vi "Process.vi"(8 "error in (no error)":errorcluster, 10 "Pound in":refnum<class "Pound.lvclass">, 11 "Qbus in":refnum<class "Qbus.lvclass">) -> (0 "error out":errorcluster)   [LabVIEW 2017, in "BurstMode.lvlib"]
doc: "The Trigger process evaluates the expressions that define when a data group enters and exits operating states. After determining the current operating state of the data goup, this process evaluates the file-collection expression for that state to determine whether to collect a file."
uses:
  <vilib>/addons/InsightCM/Devices/Shared/Cms/CmsBurstMode/BurstMode.lvlib
  <vilib>/addons/Qbus/Qbus.lvclass
  <vilib>/NI/Software Watchdog/Pound/Pound.lvclass
  <vilib>/addons/InsightCM/Devices/Shared/Cms/CmsBurstMode/controls/config.ctl
  <vilib>/addons/TimerProcess/controls/taskType.ctl
  <vilib>/addons/InsightCM/Devices/Shared/Cms/CmsBurstMode/controls/BurstModeComplete.ctl
  <vilib>/NI/Software Watchdog/Watchdog/Watchdog.lvclass
  <vilib>/addons/TraceLogger/TraceLogger.lvlib
  <vilib>/addons/InsightCM/Devices/Shared/Common/ServerComm/ServerComm.lvlib
  <vilib>/addons/InsightCM/Devices/Shared/Common/DataFlow/DataFlow.lvlib
  <vilib>/addons/InsightCM/Utilities/GlobalConfiguration/GlobalConfiguration.lvlib
  <vilib>/addons/TimerProcess/TimerProcess.lvlib
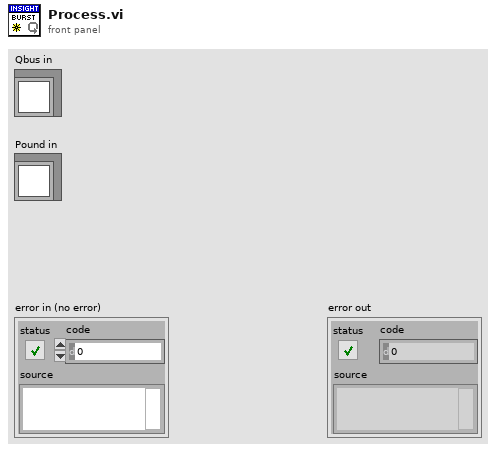
[diagram p1: front panel]
types:
  T1 = typedef "BurstMode.lvlib/config.ctl" = cluster{"Device":string, "Groups":string[], "ForceBurst":variant, "TriggerBurst":variant, "Burst Mode Count":i32, "Enabled":bool}
  T2 = typedef "TimerProcess.lvlib/taskType.ctl" = enum16{"single", "repeat"}
  T3 = typedef "BurstMode.lvlib/BurstModeComplete.ctl" = cluster{"Group":string}
  T4 = typedef "DataFlow.lvlib/Data.ctl" = cluster{"DataGroup":string, "Waveforms":T5, "Map":T6, "Type":T7}
  T5 = typedef "wfmSGL_DVR.ctl" = refnum<data-value>
  T6 = typedef "PointValueMap.lvlib/PointMap.ctl" = refnum<data-value>
  T7 = typedef "DataFlow.lvlib/Type.ctl" = enum16{"High Rate", "Low Rate", "Burst Mode"}
  T8 = typedef "Message.ctl" = cluster{"Header":T9, "Body":u8[]}
  T9 = typedef "MessageHeader.ctl" = cluster{"MessageName":string, "Timestamp":i64, "CorrelationId":string, "ContentType":string, "RoutingKey":string, "Properties":T10[]}
  T10 = typedef "KeyValuePair.ctl" = cluster{"Key":string, "Value":string}
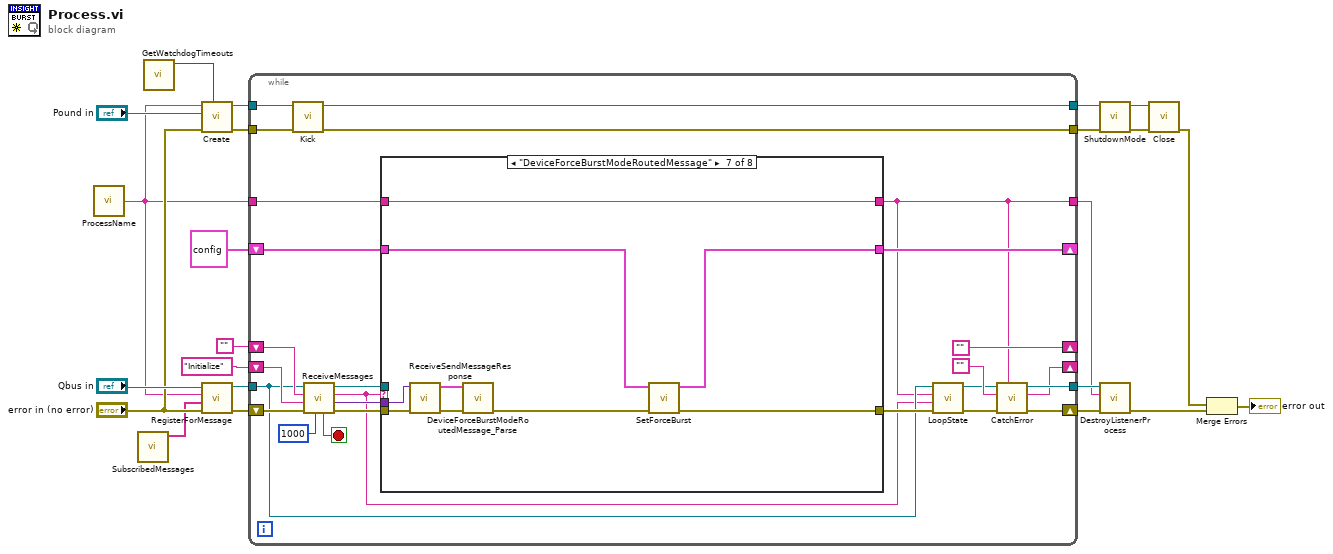
[diagram p0: block diagram]
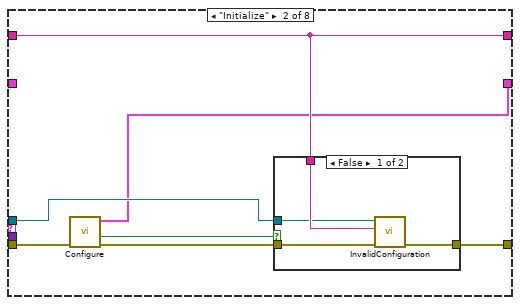
[diagram p3: hidden frame]
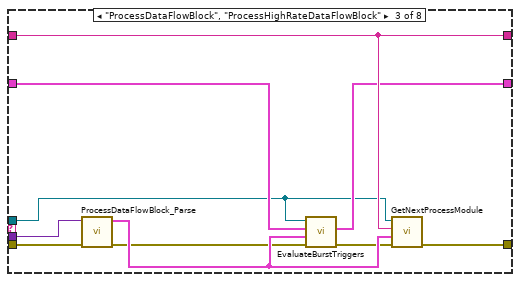
[diagram p5: hidden frame]
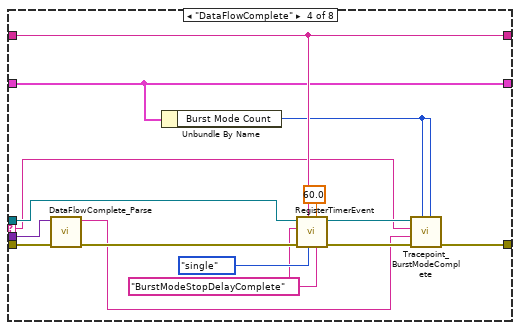
[diagram p6: hidden frame]
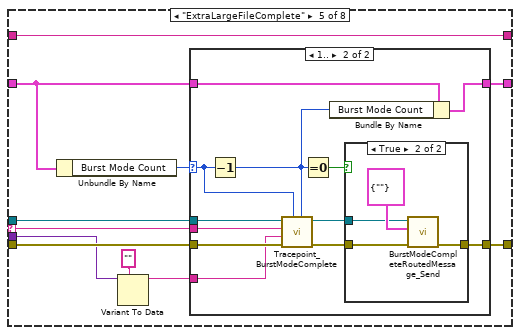
[diagram p7: hidden frame]
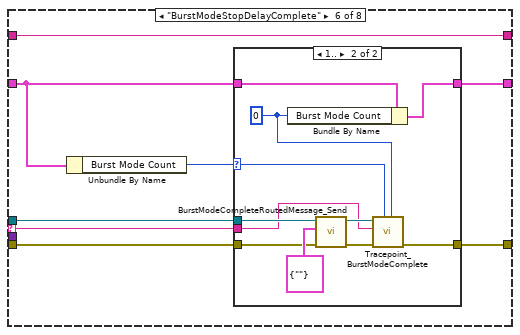
[diagram p10: hidden frame]
diagram:
  n1 = call <vilib>:"ProcessName.vi"() -> ("process name"=w3:string)  [unwired: 5 in]
  n2 = call <vilib>:"SubscribedMessages.vi"() -> ("subscribed messages"=w2:string[])  [unwired: 11 in]
  n3 = call <vilib>:"GetWatchdogTimeouts.vi"() -> ("software timeout"=w4:u32)  [unwired: 10 in, 1 out]
  n4 = call <vilib>:"Create.vi"("Execution Timeout (ms)"=w4, "error in (no error)"="error in (no error)", "Pound"="Pound in", "Name"=w3) -> ("error out"=w13:errorcluster, "Watchdog"=w12:refnum<data-value>)  [unwired: 6 in]
  n5 = call <vilib>:"RegisterForMessage.vi"("error in (no error)"="error in (no error)", "message names"=w2, "process name"=w3, "Qbus in"="Qbus in") -> ("error in (no error)"=w22:errorcluster, "Qbus out"=w21:refnum<class "Qbus.lvclass">)  [unwired: 6 in]
  n6 = while {
    shift-right: [""] -> _
    shift-left: "" -> [w47]
    tunnel: w21 -> [w33]
    tunnel: w3 -> [w35]
    tunnel: [w38] -> w18
    tunnel: [w28] -> w17
    shift-right: [w36] -> _
    shift-left: "Initialize" -> [w42]
    shift-right: [w40] -> _
    shift-left: T1 {"Device"="", "Groups"=[], "ForceBurst"=variant, "TriggerBurst"=variant, "Burst Mode Count"=0, "Enabled"=FALSE} ("config") -> [w41]
    tunnel: w13 -> [w32]
    tunnel: w12 -> [w31]
    tunnel: [w30] -> w8
    tunnel: [w29] -> w7
    shift-right: [w39] -> w20
    shift-left: w22 -> [w49]
    stop <- w48 stop-if-true
    n7 = call <vilib>:"Kick.vi"("error in (no error)"=w32, "Watchdog"=w31) -> ("error out"=w29:errorcluster, "Watchdog"=w30:refnum<data-value>)  [unwired: 8 in]
    n8 = call <vilib>:"ReceiveMessages.vi"("timeout (1000)"=1000 ("milliseconds to wait"), "error in (no error)"=w49, "priority action"=w42, "default action"=w47, "Qbus in"=w33) -> ("error out"=w46:errorcluster, "message value"=w43:variant, "action"=w27:string, "Qbus out"=w44:refnum<class "Qbus.lvclass">, "exit"=w48:bool)  [unwired: 2 in]
    n9 = case shown="\"DeviceForceBurstModeRoutedMessage\"" w27 {
      selector: w27 -> [_ _ _ w78 w95 w123 _ _]
      tunnel: w46 -> [w50 w56 w73 w88 w100 w126 w148 w150]
      tunnel: w44 -> [_ w59 w65 w87 w98 w124 _ _]
      tunnel: [w50 w58 w74 w79 w99 w125 w144 w150] -> w34
      tunnel: w43 -> [_ _ w72 w89 w92 _ w147 _]
      tunnel: w41 -> [w52 _ w70 w77 w96 w121 w146 w152]
      tunnel: [w52 w53 w69 w77 w97 w120 w145 w152] -> w40
      tunnel: [w51 w57 w71 w86 w93 w127 w149 w151] -> w28
      tunnel: w35 -> [w51 w57 w71 w86 w93 w127 w149 w151]
      frame "", Default {
      }
      frame "Initialize" {
        n10 = call <vilib>:"Configure.vi"("error in (no error)"=w56) -> ("error out"=w55:errorcluster, "valid configuration"=w54:bool, "config"=w53:T1)  [unwired: 8 in]
        n11 = case shown="False" w54 {
          tunnel: w59 -> [w61 _]
          tunnel: [w63 w64] -> w58
          tunnel: w55 -> [w60 w64]
          tunnel: w57 -> [w62 _]
          frame False {
            n12 = call <vilib>:"InvalidConfiguration.vi"("error in (no error)"=w60, "description"=w62, "Qbus in"=w61) -> ("error out"=w63:errorcluster)  [unwired: 7 in, 1 out]
          }
          frame True {
          }
        }
      }
      frame "ProcessDataFlowBlock", "ProcessHighRateDataFlowBlock" {
        n13 = call <vilib>:"ProcessDataFlowBlock_Parse.vi"("error in (no error)"=w73, "body"=w72) -> ("error out"=w67:errorcluster, "data"=w68:T4)  [unwired: 8 in]
        n14 = call <vilib>:"EvaluateBurstTriggers.vi"("error in (no error)"=w67, "data"=w68, "config"=w70, "Qbus in"=w65) -> ("error out"=w66:errorcluster, "config out"=w69:T1)  [unwired: 6 in]
        n15 = call <vilib>:"GetNextProcessModule.vi"("error in (no error)"=w66, "data"=w68, "source"=w71, "Qbus in"=w65) -> ("error out"=w74:errorcluster)  [unwired: 6 in, 1 out]
      }
      frame "DataFlowComplete" {
        w82 = "BurstModeStopDelayComplete" ("timer task name")
        n16 = call <vilib>:"DataFlowComplete_Parse.vi"("error in (no error)"=w88, "body"=w89) -> ("error out"=w85:errorcluster, "group"=w75:string)  [unwired: 8 in]
        n17 = Unbundle By Name(w77) -> ("Burst Mode Count"=w76:i32)
        n18 = call <vilib>:"RegisterTimerEvent.vi"("timer task name"=w82, "interval (sec)"=60.0, "type"=taskType."single", "process name"=w86, "error in (no error)"=w85, "callback action"=w82, "qbus in"=w87) -> ("error out"=w80:errorcluster, "qbus out"=w81:refnum<class "Qbus.lvclass">)  [unwired: 3 in]
        n19 = call <vilib>:"Tracepoint_BurstModeComplete.vi"("new count"=w76, "prev count"=w76, "error in (no error)"=w80, "group"=w75, "type"=w78, "Qbus"=w81) -> ("error out"=w79:errorcluster)  [unwired: 4 in, 1 out]
      }
      frame "ExtraLargeFileComplete" {
        n20 = Unbundle By Name(w96) -> ("Burst Mode Count"=w94:i32)
        n21 = Variant To Data(type="", Variant=w92) -> (data=w90:string)  [unwired: 1 in, 1 out]
        n22 = case shown="1.." w94 {
          selector: w94 -> [_ w104]
          tunnel: w100 -> [w101 w108]
          tunnel: [w101 w114] -> w99
          tunnel: w98 -> [_ w110]
          tunnel: w95 -> [_ w105]
          tunnel: w96 -> [w102 w112]
          tunnel: [w102 w111] -> w97
          tunnel: w90 -> [_ w106]
          frame 0, Default {
          }
          frame 1.. {
            n23 = Decrement(x=w104) -> (x-1=w103:i32)
            n24 = call <vilib>:"Tracepoint_BurstModeComplete.vi"("new count"=w103, "prev count"=w104, "error in (no error)"=w108, "group"=w106, "type"=w105, "Qbus"=w110) -> ("error out"=w107:errorcluster, "Qbus out"=w109:refnum<class "Qbus.lvclass">)  [unwired: 4 in]
            n25 = Equal To 0?(x=w103) -> (x = 0?=w113:bool)
            n26 = Bundle By Name(cluster=w112, "Burst Mode Count"=w103) -> (w111:T1)
            n27 = case shown="True" w113 {
              tunnel: w107 -> [w115 w118]
              tunnel: [w115 w116] -> w114
              tunnel: w109 -> [_ w117]
              frame False {
              }
              frame True {
                n28 = call <vilib>:"BurstModeCompleteRoutedMessage_Send.vi"("error in (no error)"=w118, "BurstModeComplete"=T3 {"Group"=""}, "Qbus in"=w117) -> ("error out"=w116:errorcluster)  [unwired: 7 in, 1 out]
              }
            }
          }
        }
      }
      frame "BurstModeStopDelayComplete" {
        n29 = Unbundle By Name(w121) -> ("Burst Mode Count"=w122:i32)
        n30 = case shown="1.." w122 {
          selector: w122 -> [_ w131]
          tunnel: w126 -> [w128 w138]
          tunnel: [w128 w137] -> w125
          tunnel: w124 -> [_ w136]
          tunnel: w123 -> [_ w134]
          tunnel: w121 -> [w129 w133]
          tunnel: [w129 w132] -> w120
          frame 0, Default {
          }
          frame 1.. {
            w130 = 0 ("Burst Mode Count")
            n31 = Bundle By Name(cluster=w133, "Burst Mode Count"=w130) -> (w132:T1)
            n32 = call <vilib>:"BurstModeCompleteRoutedMessage_Send.vi"("error in (no error)"=w138, "BurstModeComplete"=T3 {"Group"=""}, "Qbus in"=w136) -> ("error out"=w139:errorcluster, "Qbus out"=w135:refnum<class "Qbus.lvclass">)  [unwired: 7 in]
            n33 = call <vilib>:"Tracepoint_BurstModeComplete.vi"("new count"=w130, "prev count"=w131, "error in (no error)"=w139, "type"=w134, "Qbus"=w135) -> ("error out"=w137:errorcluster)  [unwired: 5 in, 1 out]
          }
        }
      }
      frame "DeviceForceBurstModeRoutedMessage" {
        n34 = call <vilib>:"ReceiveSendMessageResponse.vi"("error in (no error)"=w148, "body"=w147) -> ("error out"=w142:errorcluster, "message"=w143:T8)  [unwired: 6 in, 2 out]
        n35 = call <vilib>:"DeviceForceBurstModeRoutedMessage_Parse.vi"("error in (no error)"=w142, "Message"=w143) -> ("error out"=w141:errorcluster)  [unwired: 7 in, 2 out]
        n36 = call <vilib>:"SetForceBurst.vi"("error in (no error)"=w141, "config"=w146) -> ("error out"=w144:errorcluster, "config out"=w145:T1)  [unwired: 8 in]
      }
      frame "Exit" {
      }
    }
    n37 = call <vilib>:"LoopState.vi"("error in (no error)"=w34, "loop action"=w27, "process name"=w28, "Qbus in"=w33) -> ("error out"=w25:errorcluster, "Qbus out"=w24:refnum<class "Qbus.lvclass">)  [unwired: 6 in]
    n38 = call <vilib>:"CatchError.vi"("source"=w28, "error in (no error)"=w25, "next action in"="", "Qbus in"=w24) -> ("error out"=w39:errorcluster, "next action out"=w36:string, "Qbus out"=w38:refnum<class "Qbus.lvclass">)  [unwired: 5 in]
  }
  n39 = call <vilib>:"ShutdownMode.vi"("error in (no error)"=w7, "Watchdog"=w8) -> ("error out"=w10:errorcluster, "Watchdog"=w9:refnum<data-value>)  [unwired: 8 in]
  n40 = call <vilib>:"DestroyListenerProcess.vi"("error in (no error)"=w20, "process name"=w17, "Qbus in"=w18) -> ("error in (no error)"=w19:errorcluster)  [unwired: 7 in, 1 out]
  n41 = call <vilib>:"Close.vi"("error in (no error)"=w10, "Watchdog"=w9) -> ("error out"=w5:errorcluster)  [unwired: 9 in]
  n42 = Merge Errors(w5, w19) -> (→"error out":errorcluster)
